vi "Drive_Normalize_and_Native_Units.vi"(4 "BR":dbl, 5 "BL":dbl, 6 "FR":dbl, 7 "FL":dbl) -> (0 "BR_Out":dbl, 1 "BL_Out":dbl, 2 "FR_Out":dbl, 3 "FL_Out":dbl)   [LabVIEW 2018]
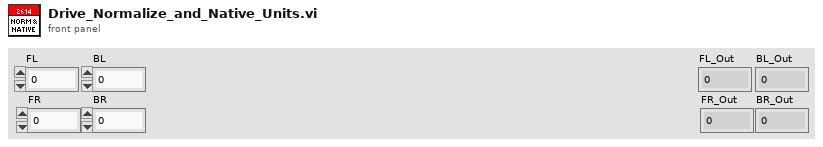
[diagram p1: front panel]
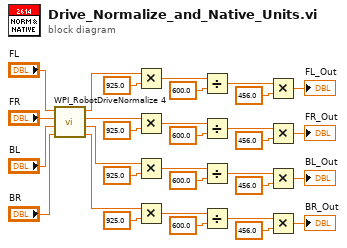
[diagram p0: block diagram]
diagram:
  n1 = call <vilib>:"WPI_RobotDriveNormalize 4.vi"("D"="BR", "C"="BL", "B"="FR", "A"="FL") -> ("D'"=w32:dbl, "C'"=w31:dbl, "B'"=w30:dbl, "A'"=w29:dbl)
  n2 = Multiply(x=w29, y=925.0) -> (x*y=w12:dbl)
  n3 = Multiply(x=w30, y=925.0) -> (x*y=w15:dbl)
  n4 = Multiply(x=w31, y=925.0) -> (x*y=w22:dbl)
  n5 = Multiply(x=w32, y=925.0) -> (x*y=w25:dbl)
  n6 = Divide(x=w12, y=600.0) -> (x/y=w9:dbl)
  n7 = Divide(x=w15, y=600.0) -> (x/y=w18:dbl)
  n8 = Divide(x=w22, y=600.0) -> (x/y=w19:dbl)
  n9 = Divide(x=w25, y=600.0) -> (x/y=w28:dbl)
  n10 = Multiply(x=w9, y=456.0) -> (x*y=→"FL_Out":dbl)
  n11 = Multiply(x=w18, y=456.0) -> (x*y=→"FR_Out":dbl)
  n12 = Multiply(x=w19, y=456.0) -> (x*y=→"BL_Out":dbl)
  n13 = Multiply(x=w28, y=456.0) -> (x*y=→"BR_Out":dbl)
